vi "TMCM351-goZero.vi"(4 "motor":u8(ring) items=["x", "y", "z"], 5 "错误输入":errorcluster caption="错误输入（无错误）", 8 "com in":refnum<visa-resource-name>) -> (0 "错误输出":errorcluster, 3 "com out":refnum<visa-resource-name>)   [LabVIEW 2018]
uses:
  module_param.vi
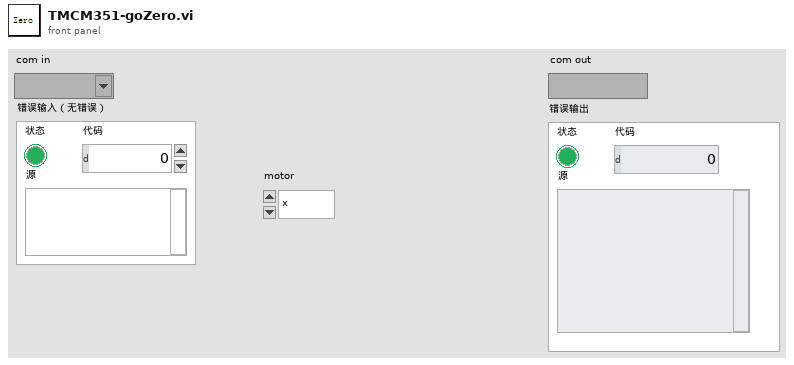
[diagram p1: front panel]
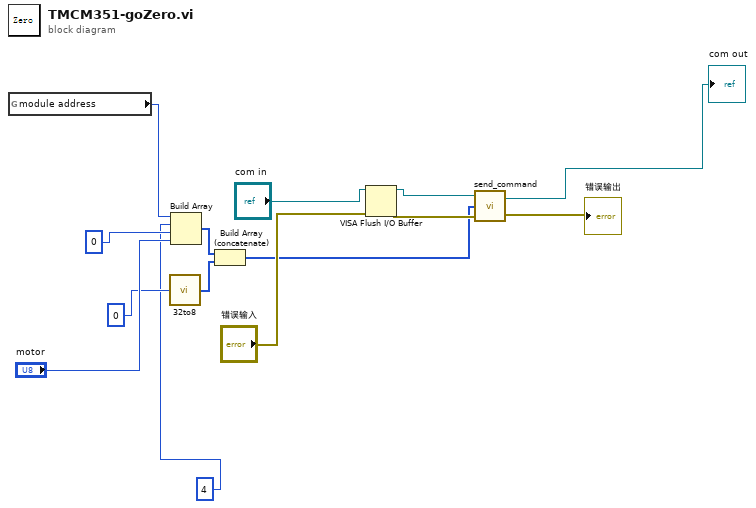
[diagram p0: block diagram]
diagram:
  n1 = global read "module_param.vi" "module address"() -> (w13:u8)
  n2 = call "32to8.vi"("32data_in"=0) -> ("8Array"=w4:u8[])
  n3 = Build Array(w13, u8 4 ("元素"), u8 0, "motor") -> (w5:u8[])
  n4 = Build Array (concatenate)(w5, w4) -> (w3:u8[])
  n5 = VISA Flush I/O Buffer(VISA resource name="com in", error in (no error)="错误输入") -> (VISA resource name out=w9:refnum<visa-resource-name>, error out=w8:errorcluster)  [unwired: 1 in]
  n6 = call "send_command.vi"("错误输入"=w8, 3:w3, "com in"=w9) -> ("错误输出"=→"错误输出":errorcluster, "com out"=→"com out":refnum<visa-resource-name>)
